vi "Untitled 1.vi"() -> ()   [LabVIEW 2019]
uses:
  <vilib>/rvi/Emulation/niFpgaGetClockAttributes.vi
  <vilib>/rvi/Emulation/niFpgaSctlEmulationGetInTimedLoop.vi
  <vilib>/rvi/Emulation/niFpgaEmulationReportErrorSimple.vi
  <vilib>/rvi/Emulation/niFpgaCriticalErrorInLSC.vi
panel:
  in  "Trigger Condition":bool
  out "LED":bool
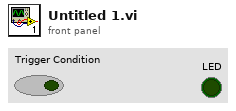
[diagram p1: front panel]
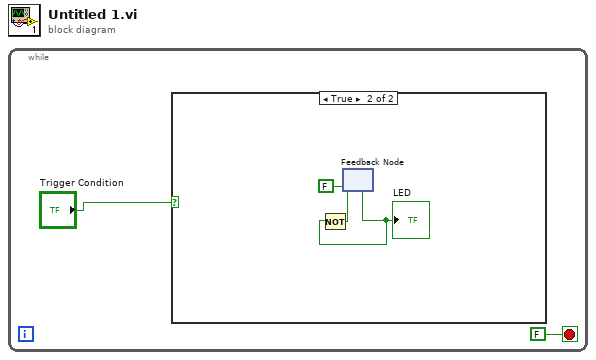
[diagram p0: block diagram]
diagram:
  n1 = while {
    stop <- FALSE stop-if-true
    n2 = case shown="True" "Trigger Condition" {
      frame False {
      }
      frame True {
        n3 = feedback #1(FALSE) -> (w4:bool)
        "LED" <- w4
        n4 = Not(x=w4) -> (.not. x?=w5:bool)
        n5 = feedback-in #1(w5) -> ()
      }
    }
  }
